vi "Update Data.vi"(0 "DATA in":T1, 7 "Value":dbl) -> (4 "DATA iout":T1)   [LabVIEW 2019, in "OscillationDetector.lvclass"]
uses:
  OscillationDetector.lvclass
  DATA Oscill.ctl
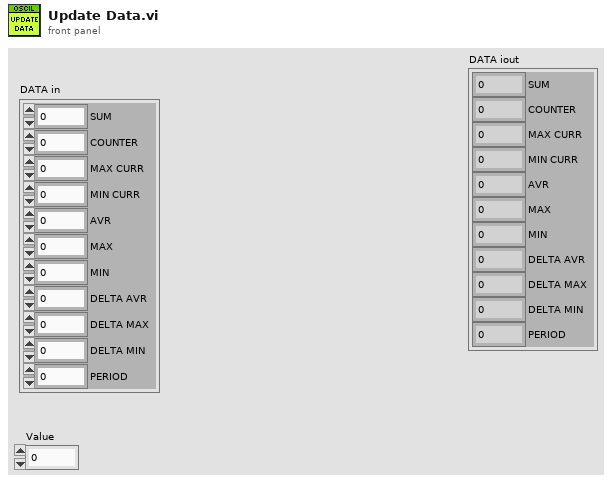
[diagram p1: front panel]
types:
  T1 = typedef "DATA Oscill.ctl" = cluster{"SUM":dbl, "COUNTER":dbl, "MAX CURR":dbl, "MIN CURR":dbl, "AVR":dbl, "MAX":dbl, "MIN":dbl, "DELTA AVR":dbl, "DELTA MAX":dbl, "DELTA MIN":dbl, "PERIOD":dbl}
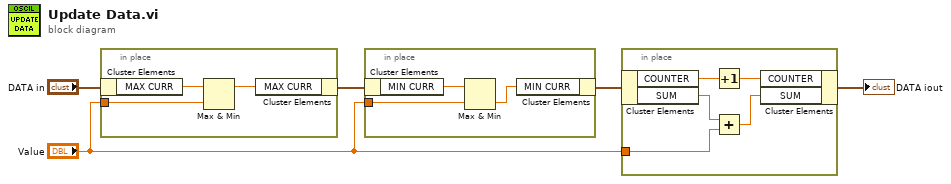
[diagram p0: block diagram]
diagram:
  n1 = in-place {
    in-place-border: "Value" -> [w7]
    n2 = in-place-cluster #1("DATA in") -> ("MAX CURR"=w8:dbl)
    n3 = Max & Min(x=w8, y=w7) -> (max(x,y)=w6:dbl)  [unwired: 1 out]
    n4 = in-place-cluster #1("MAX CURR"=w6) -> (w5:T1)
  }
  n5 = in-place {
    in-place-border: "Value" -> [w11]
    n6 = in-place-cluster #2(w5) -> ("MIN CURR"=w10:dbl)
    n7 = Max & Min(x=w10, y=w11) -> (min(x,y)=w9:dbl)  [unwired: 1 out]
    n8 = in-place-cluster #2("MIN CURR"=w9) -> (w4:T1)
  }
  n9 = in-place {
    in-place-border: "Value" -> [w16]
    n10 = in-place-cluster #3(w4) -> ("COUNTER"=w13:dbl, "SUM"=w15:dbl)
    n11 = Increment(x=w13) -> (x+1=w12:dbl)
    n12 = Add(x=w15, y=w16) -> (x+y=w14:dbl)
    n13 = in-place-cluster #3("COUNTER"=w12, "SUM"=w14) -> (→"DATA iout":T1)
  }
